vi "SetControlToDefault.vi"(8 "error in (no error)":errorcluster, 10 "Control Array In":string[](array[string]), 11 "CtlLookup In":T1) -> (0 "error in (no error) Out":errorcluster, 3 "CtlLookup Out":T1)   [LabVIEW 2018, in "CtlReferences_API.lvlib"]
uses:
  CtlReferences_API.lvlib
  TypeDefs/CtlLookup.ctl
  CtlReferences.lvclass
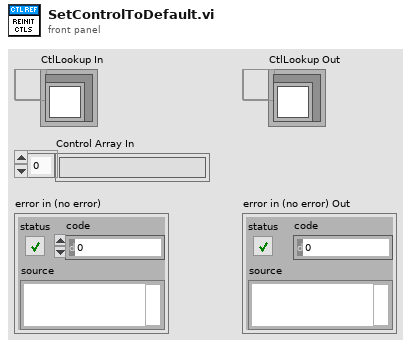
[diagram p1: front panel]
types:
  T1 = typedef "CtlReferences.lvlib/CtlReferences.lvclass/CtlLookup.ctl" = refnum<data-value>
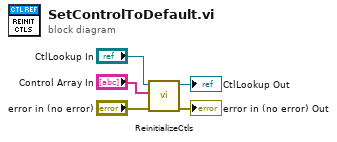
[diagram p0: block diagram]
diagram:
  n1 = call "ReinitializeCtls.vi"("error in (no error)"="error in (no error)", "Control Array In"="Control Array In", "CtlLookup In"="CtlLookup In") -> ("error in (no error) Out"=→"error in (no error) Out":errorcluster, "CtlLookup Out"=→"CtlLookup Out":T1)  [unwired: 7 in]
